vi "DllFxpNaturalLogarithmTemp.vi"(6 "ready for output":bool, 9 "input valid":bool, 11 "x":fxp<+/-,64,32>) -> (1 "output valid":bool, 3 "ln":fxp<+,1,1>, 4 "ready for input":bool, 5 "undefined":bool)   [LabVIEW 2017]
uses:
  <vilib>/rvi/FXPMathLib/FxpLn/subVIs/nifxpmath_NaturalLogarithm_SimConfig.ctl
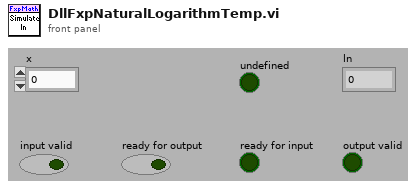
[diagram p1: front panel]
types:
  T1 = typedef "nifxpmath_NaturalLogarithm_SimConfig.ctl" = cluster{"kXLen":u16, "kLnLen":u16, "kInputRegister":bool, "kOutputRegister":bool, "kLowLimit":u64, "kPrecision":u16, "kIteration":u16, "QuantiMode":u16, "HandShake":bool, "CycleLimit":u16, "StrictLimit":bool}
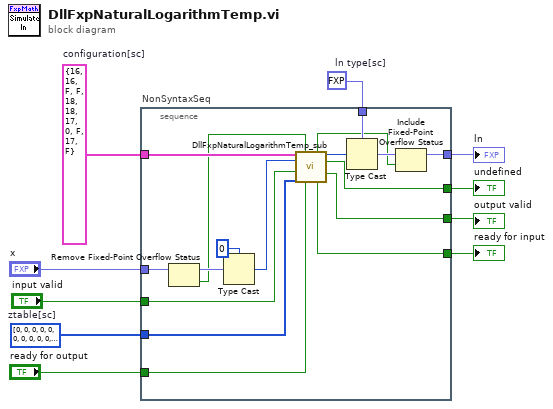
[diagram p0: block diagram]
diagram:
  w1 = T1 {"kXLen"=16, "kLnLen"=16, "kInputRegister"=FALSE, "kOutputRegister"=FALSE, "kLowLimit"=18, "kPrecision"=18, "kIteration"=17, "QuantiMode"=0, "HandShake"=FALSE, "CycleLimit"=17, "StrictLimit"=FALSE}  # configuration[sc]
  w8 = fxp<+,1,1> 0.0  # ln type[sc]
  w9 = u64[] [0, 0, 0, 0, 0, 0, 0, 0, 0, 0, 0, 0, 0, 0, 0, 0]  # ztable[sc]
  n1 = stacked-sequence "NonSyntaxSeq" {
    tunnel: w8 -> [w26]
    tunnel: w9 -> [w19]
    tunnel: "x" -> [w25]
    tunnel: w1 -> [w23]
    tunnel: "input valid" -> [w20]
    tunnel: "ready for output" -> [w18]
    tunnel: [w14] -> w4
    tunnel: [w13] -> w3
    tunnel: [w12] -> w5
    tunnel: [w11] -> w2
    frame #0 {
      n2 = Remove Fixed-Point Overflow Status(3:w25) -> (0:w21:bool, 1:w24:fxp<+/-,64,32>)
      n3 = Type Cast(type=u64 0, x=w24) -> (*(type *) &x=w22:u64)
      n4 = call <vilib>:"DllFxpNaturalLogarithmTemp_sub.vi"("configuration[sc]"=w23, "x ovfl status"=w21, "x"=w22, "input valid"=w20, "ztable"=w19, "ready for output"=w18) -> ("ln ovfl status"=w15:bool, "ln"=w17:u64, "undefined"=w14:bool, "output valid"=w13:bool, "ready for input"=w11:bool)  [unwired: 5 out]
      n5 = Type Cast(type=w26, x=w17) -> (*(type *) &x=w16:fxp<+,1,1>)
      n6 = Include Fixed-Point Overflow Status(2:w15, 3:w16) -> (1:w12:fxp<+,1,1>)
    }
  }
  "ln" <- w5
  "output valid" <- w3
  "ready for input" <- w2
  "undefined" <- w4
